vi "Engine_test.vi"() -> ()   [LabVIEW 2026]
panel:
  out "error out":errorcluster
  out "valid?":bool
  out "Rs (Ohm/sq)":dbl
  in  "Keithley VISA":refnum<visa-resource-name>
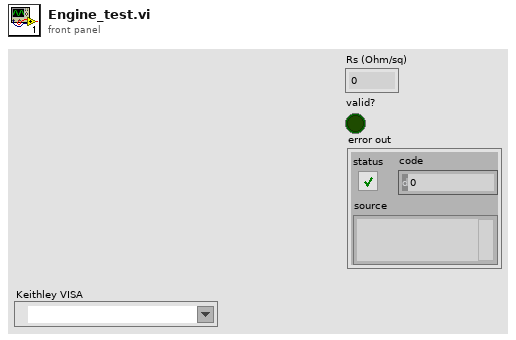
[diagram p1: front panel]
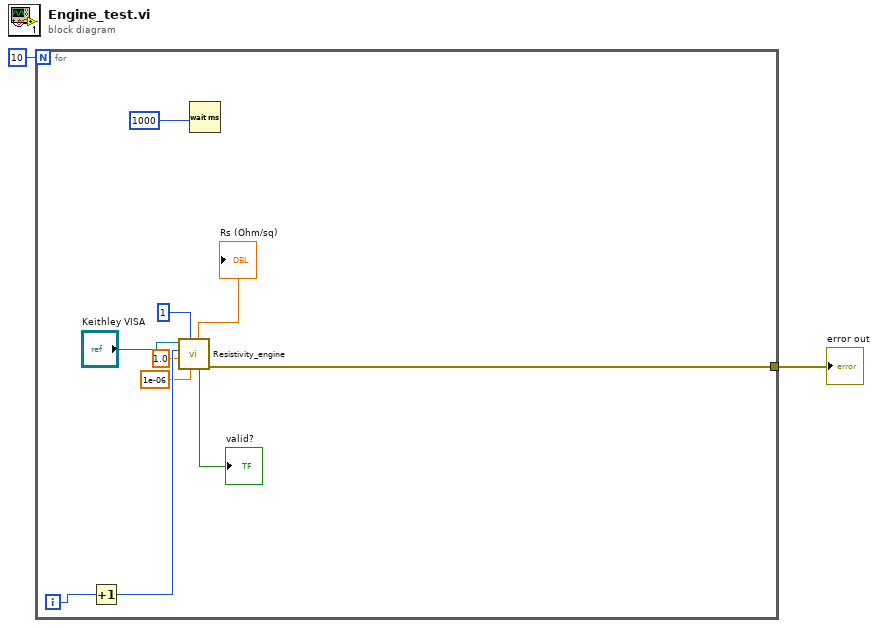
[diagram p0: block diagram]
diagram:
  n1 = for {
    N: 10 -> [_]
    tunnel: [w5] -> w1
    i -> [w12]
    n2 = Increment(x=w12) -> (x+1=w11:i32)
    n3 = call "Resistivity_engine.vi"("I (A)"=1e-06, "M"=1, "GPC (A/cycle)"=1.0, "N (cycle)"=w11, "Keithley VISA"="Keithley VISA") -> ("error out"=w5:errorcluster, "valid?"=→"valid?":bool, "Rs (Ohm/sq)"=→"Rs (Ohm/sq)":dbl)  [unwired: 2 in, 2 out]
    n4 = Wait (ms)(milliseconds to wait=u32 1000 ("millisecond timer value")) -> ()  [unwired: 1 out]
  }
  "error out" <- w1
